vi "EMV Determine UL and LL Spec.vi"(7 "Position?":bool, 8 "error in (no error)":errorcluster, 11 "Input":T1) -> (0 "error out":errorcluster, 3 "Output":T1)   [LabVIEW 2016]
uses:
  type defs/EMV Flow Stop Detection.ctl
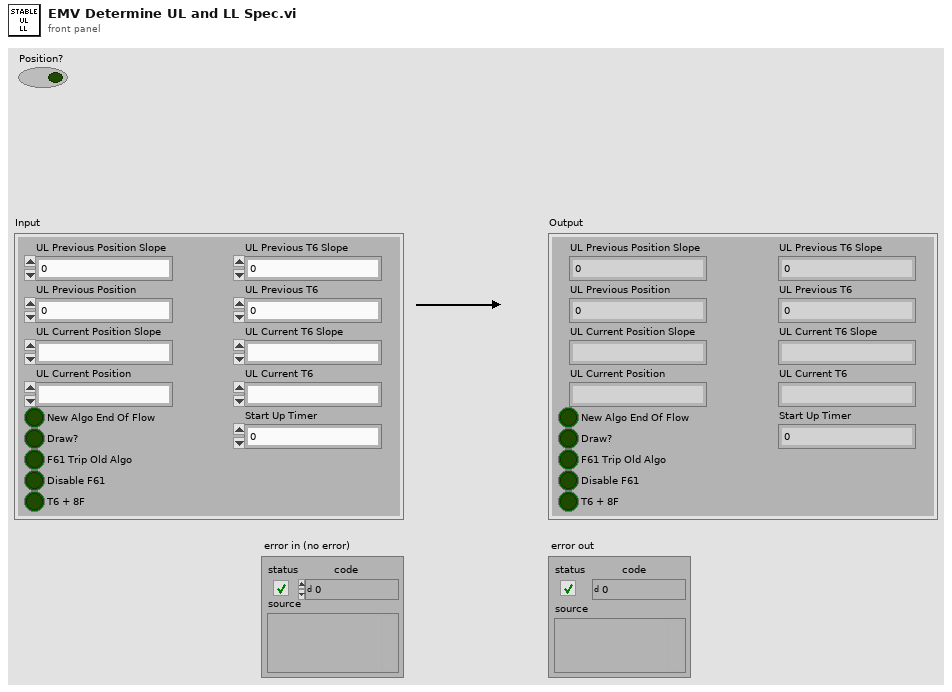
[diagram p1: front panel]
types:
  T1 = typedef "EMV Flow Stop Detection.ctl" = cluster{"UL Previous Position Slope":dbl, "UL Previous T6 Slope":dbl, "UL Previous Position":dbl, "UL Previous T6":dbl, "UL Current Position":dbl, "UL Current Position Slope":dbl, "UL Current T6":dbl, "UL Current T6 Slope":dbl, "New Algo End Of Flow":bool, "Start Up Timer":dbl, "Draw?":bool, "Disable F61":bool, "F61 Trip Old Algo":bool, "T6 + 8F":bool}
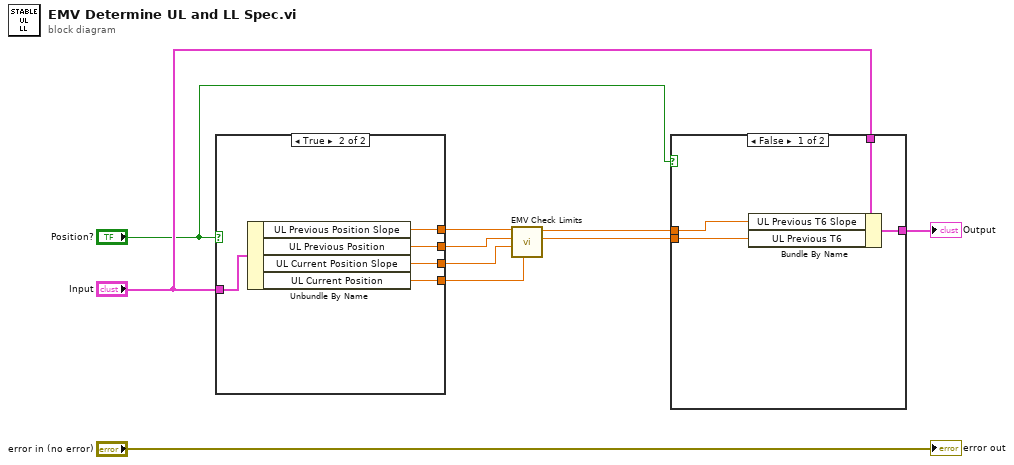
[diagram p0: block diagram]
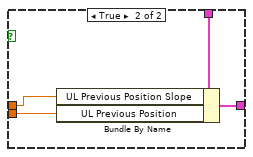
[diagram p2: hidden frame]
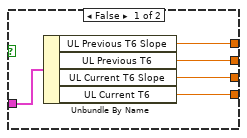
[diagram p3: hidden frame]
diagram:
  n1 = case shown="True" "Position?" {
    tunnel: [w12 w17] -> w2
    tunnel: [w14 w20] -> w6
    tunnel: "Input" -> [w15 w19]
    tunnel: [w13 w18] -> w3
    tunnel: [w11 w16] -> w1
    frame False {
      n2 = Unbundle By Name(w15) -> ("UL Previous T6 Slope"=w13:dbl, "UL Previous T6"=w14:dbl, "UL Current T6 Slope"=w12:dbl, "UL Current T6"=w11:dbl)
    }
    frame True {
      n3 = Unbundle By Name(w19) -> ("UL Previous Position Slope"=w18:dbl, "UL Previous Position"=w20:dbl, "UL Current Position Slope"=w17:dbl, "UL Current Position"=w16:dbl)
    }
  }
  n4 = call "EMV Check Limits.vi"("Current Position"=w1, "Current Position Slope"=w2, "Previous Position"=w6, "Previous Position Slope"=w3) -> ("Position"=w5:dbl, "Slope Output"=w4:dbl)  [unwired: 5 in, 1 out]
  n5 = case shown="False" "Position?" {
    tunnel: w5 -> [w22 w28]
    tunnel: w4 -> [w21 w25]
    tunnel: [w24 w27] -> w9
    tunnel: "Input" -> [w23 w26]
    frame False {
      n6 = Bundle By Name(cluster=w23, "UL Previous T6 Slope"=w21, "UL Previous T6"=w22) -> (w24:T1)
    }
    frame True {
      n7 = Bundle By Name(cluster=w26, "UL Previous Position Slope"=w25, "UL Previous Position"=w28) -> (w27:T1)
    }
  }
  "Output" <- w9
  "error out" <- "error in (no error)"
